vi "Caption Test.vi"() -> ()   [LabVIEW 2020, in "UI Controls Manager.lvlib"]
uses:
  UI Controls Manager.lvlib
  uiControlsMgr.lvclass
panel:
  out "0007":bool caption="MAIS LONGO"
  out "0006":bool caption="PARTIDA"
  out "0008":bool caption="REPETE"
  in  "0005":dbl(slide) caption="HABILIDADE" scale=0.0..10.0
  in  "0004":bool caption="Amarelo"
  in  "0003":bool caption="Verde"
  in  "0002":bool caption="Azul"
  in  "0001":bool caption="Vermelho"
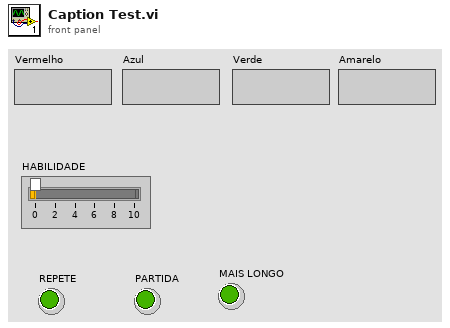
[diagram p1: front panel]
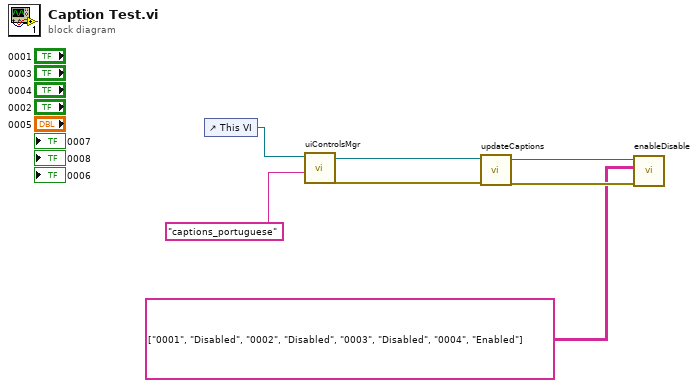
[diagram p0: block diagram]
diagram:
  n1 = control-ref of="This VI"() -> (w1:refnum<vi>)
  n2 = call "uiControlsMgr.vi"("Captions File"="captions_portuguese", "VI reference"=w1) -> ("error out"=w6:errorcluster, "uiControlsMgr out"=w7:refnum<class "uiControlsMgr.lvclass">)  [unwired: 8 in]
  n3 = call "updateCaptions.vi"("error in (no error)"=w6, "uiControlsMgr in"=w7) -> ("error out"=w3:errorcluster, "uiControlsMgr out"=w4:refnum<class "uiControlsMgr.lvclass">)  [unwired: 8 in]
  n4 = call "enableDisable.vi"("error in (no error)"=w3, "Controls - Status"=string[][] [["0001", "Disabled"], ["0002", "Disabled"], ["0003", "Disabled"], ["0004", "Enabled"]], "uiControlsMgr in"=w4) -> ()  [unwired: 7 in, 2 out]
